vi "SCMP - Run Cbk check lyot range.vi"(8 "error in (no error)":errorcluster) -> (0 "error out":errorcluster, 3 "Stop Cookbook":bool)   [LabVIEW 2014]
panel:
  in  "Cancel":bool
  in  "Continue":bool
  # "Lyot Filter Temperature is out of the interval\n                    34.9900-35.0100 °C"
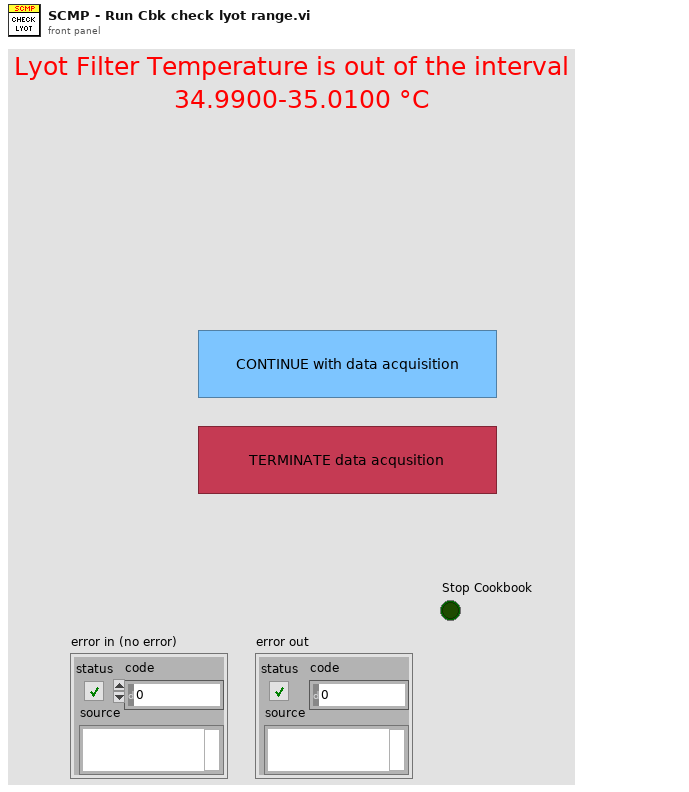
[diagram p1: front panel]
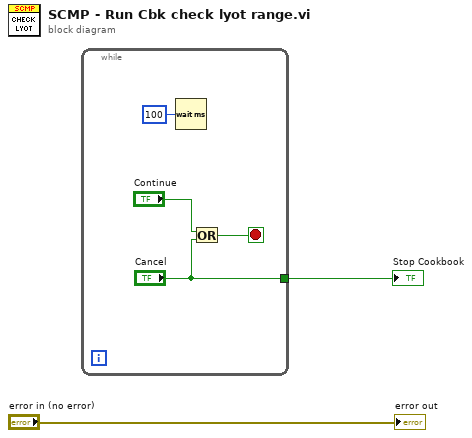
[diagram p0: block diagram]
diagram:
  n1 = while {
    tunnel: ["Cancel"] -> w1
    stop <- w4 stop-if-true
    n2 = Wait (ms)(milliseconds to wait=u32 100) -> ()  [unwired: 1 out]
    n3 = Or(x="Continue", y="Cancel") -> (x .or. y?=w4:bool)
  }
  "Stop Cookbook" <- w1
  "error out" <- "error in (no error)"
